vi "Create Subscriber.vi"(8 "error in (no error)":errorcluster, 9 "Default Value":u64, 10 "Name":string, 11 "CIFTag in":refnum<class "CIFTagU64.lvclass">) -> (0 "error out":errorcluster, 3 "CIFTag out":refnum<class "CIFTagU64.lvclass">)   [LabVIEW 2021, in "CIFTagU64.lvclass"]
uses:
  CIFTagU64.lvclass
  D:/dev/CIF-LVCore/src/CIFUtilities/CIFChannels/CIFChannels.lvclass
  D:/dev/CIF-LVCore/src/Channels/CIFTag/CIFTag/CIFTag.lvclass
  CIFUtilities/CIFChannels/Typedef/Direction.ctl
  CIFUtilities/CIFChannels/Typedef/Disconnect Behavior.ctl
  CIFUtilities/CIFChannels/Typedef/Channel State.ctl
  CIFUtilities/CIFChannels/CIFChannels.lvclass/CIFChannels.ctl
  CIFTagU64.lvclass/CIFTagU64.ctl
  CIFTag/CIFTag.lvclass/CIFTag.ctl
  175b5bb0-395a-4b4a-8cf4-aadf4605253d.vi
  72532a7b-835d-4d7a-8c97-ceeadf54b86e.vi
  CIFUtilities/CIFChannels/Accessors/Write Channel State.vi
  CIFTag/Accessors/Write CIF Channel.vi
  CIFUtilities/CIFChannels/Accessors/Write Channel Class.vi
  CIFUtilities/CIFChannels/Accessors/Write Direction.vi
  CIFUtilities/CIFChannels/Accessors/Write Disconnect Behavior.vi
  CIFUtilities/CIFChannels/Accessors/Write Name.vi
  <vilib>/CIFChannels/SubVIs/Add Error.vi
  175b5bb0-395a-4b4a-8cf4-aadf4605253d.vi/c28b0ead-42ad-4072-80a2-aca7f2bd7ce3.vi
  <vilib>/CIFChannels/SubVIs/CIFServices Fill In Error Info Ex.vi
  <vilib>/CIFChannels/SubVIs/Get dll Path.vi
  72532a7b-835d-4d7a-8c97-ceeadf54b86e.vi/4bc1c15b-36ab-481f-b8dd-c64075ce723a.vi
  <vilib>/CIFChannels/SubVIs/Append Error Location.vi
  CIFUtilities/CIFChannels/CIFChannels.lvclass
  D:/dev/CIF-LVCore/src/Channels/CIFTag/U64/CIFTagU64.lvclass
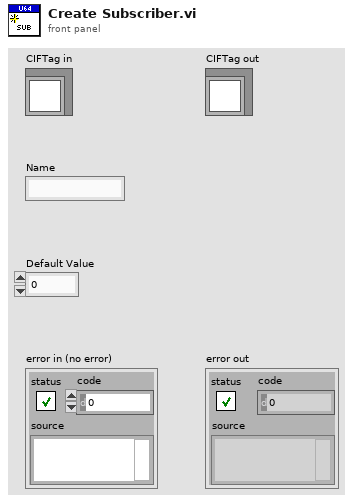
[diagram p1: front panel]
types:
  T1 = typedef "CIFChannels.lvclass/Channel State.ctl" = enum16{"Creating", "Disconnected", "Connecting", "Connected", "Destroying"}
  T2 = typedef "CIFChannels.lvclass/Disconnect Behavior.ctl" = enum16{"Default value", "Last value", "Error with default"}
  T3 = typedef "CIFChannels.lvclass/Direction.ctl" = enum16{"Publisher", "Subscriber"}
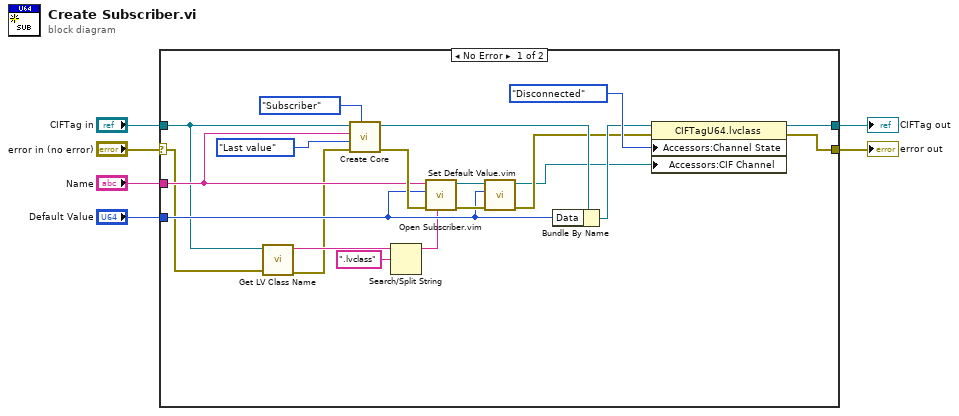
[diagram p0: block diagram]
diagram:
  n1 = case shown="No Error" "error in (no error)" {
    selector: "error in (no error)" -> [w9 w28]
    tunnel: [w23 w28] -> w4
    tunnel: [w19 w27] -> w5
    tunnel: "CIFTag in" -> [w8 w27]
    tunnel: "Name" -> [w13 _]
    tunnel: "Default Value" -> [w14 _]
    frame No Error {
      n2 = call <vilib>:"Get LV Class Name.vi"("error in (no error)"=w9, "object"=w8) -> ("error out"=w7:errorcluster, "class name"=w12:string)  [unwired: 8 in]
      n3 = call "Create Core.vi"("Direction"=Direction."Subscriber", "error in (no error)"=w7, "Disconnect Behavior"=Disconnect_Behavior."Last value", "Name"=w13, "CIFChannels in"=w8) -> ("error out"=w22:errorcluster, "CIFChannels out"=w21:refnum<class "CIFTagU64.lvclass">)  [unwired: 5 in]
      n4 = Search/Split String(string=w12, search string/char (-)=".lvclass") -> (substring before match=w10:string)  [unwired: 1 in, 2 out]
      n5 = call "Open Subscriber.vim"("Channel Type Description"=w10, "error in"=w22, "Input Type"=w14, "Channel Name"=w13) -> ("error out"=w18:errorcluster, "CIF Channel"=w17:refnum<k21>)  [unwired: 6 in]
      n6 = call "Set Default Value.vim"("error in"=w18, "Data in"=w14, "CIF Channel in"=w17) -> ("error out"=w16:errorcluster, "CIF Channel out"=w15:refnum<k21>)  [unwired: 7 in]
      n7 = Bundle By Name(cluster=w21, "Data"=w14) -> (w20:refnum<class "CIFTagU64.lvclass">)
      n8 = property class="CIFTagU64.lvclass"(reference=w20, error in=w16, "Accessors:Channel State"=Channel_State."Disconnected" ("Channel State"), "Accessors:CIF Channel"=w15) -> (reference out=w19:refnum<class "CIFTagU64.lvclass">, error out=w23:errorcluster)
    }
    frame Error {
    }
  }
  "error out" <- w4
  "CIFTag out" <- w5
